vi "FGV_REWORK_destination_selector.vi"(4 "REWORK_commit":refnum<vi>, 6 "REWORK_destination":refnum<vi>, 7 "options":T1, 8 "error_in":errorcluster, 11 "input":variant) -> (0 "error_out":errorcluster, 3 "output":variant)   [LabVIEW 2019]
uses:
  FGV_REWORK_destination_selector.ctl
  _misc/AULocalize/SubVIs/Get Localized Phrase Compact Interface 0D.vi
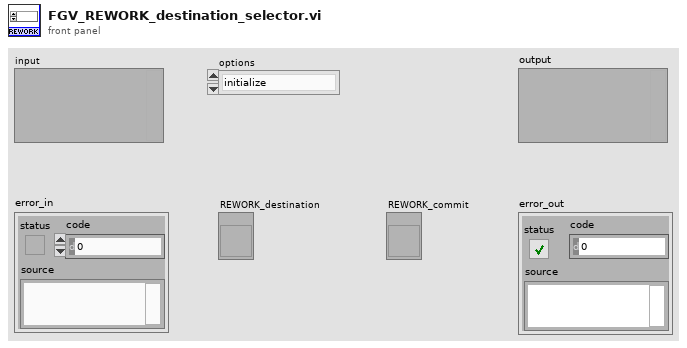
[diagram p1: front panel]
types:
  T1 = typedef "FGV_REWORK_destination_selector.ctl" = enum16{"initialize", "set_values", "display_values", "set_new_login", "enable", "disable", "disable_gray", "get_rework_to", "clear"}
  T2 = enum8{"Enabled", "Disabled", "Disabled and Grayed Out"}
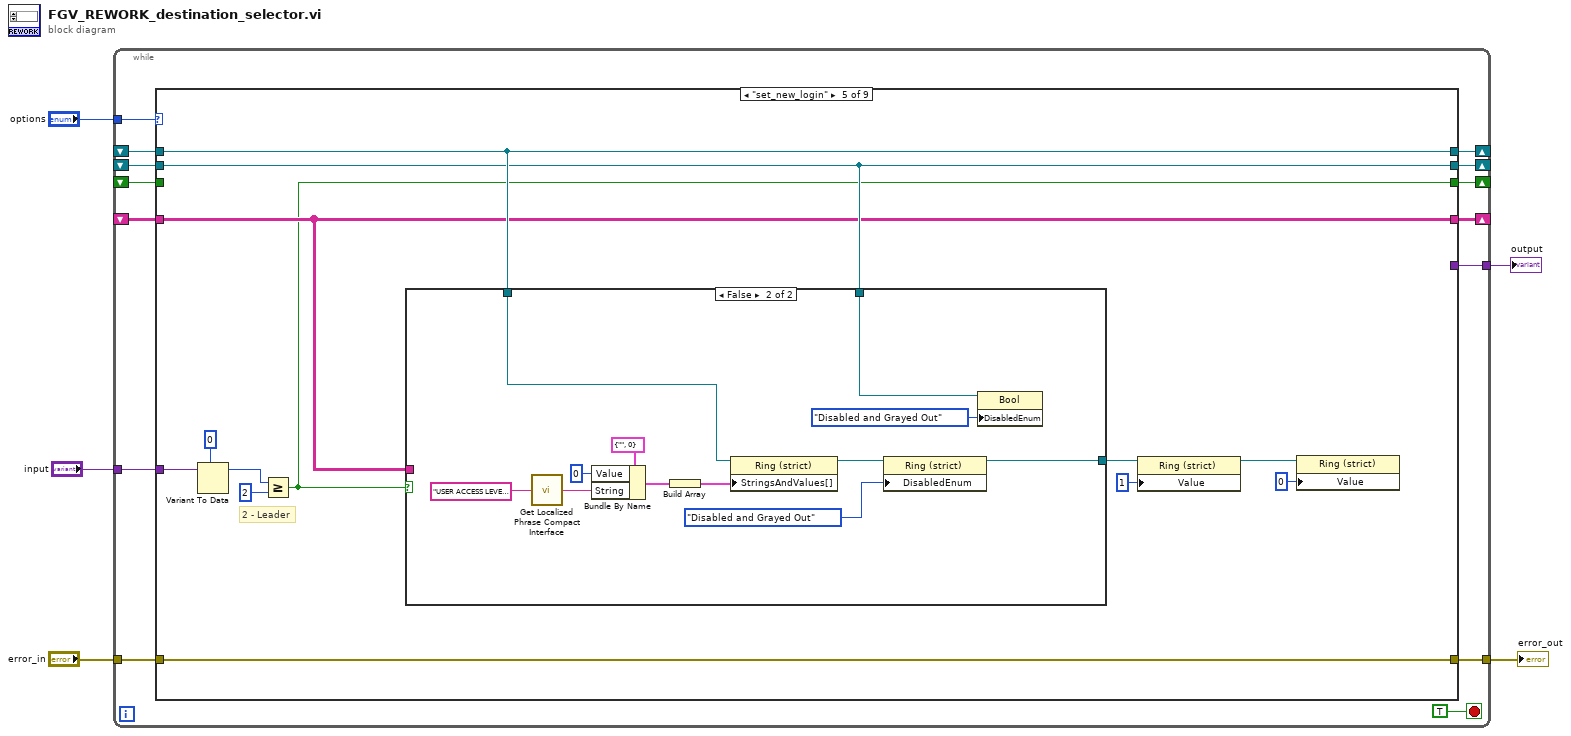
[diagram p0: block diagram]
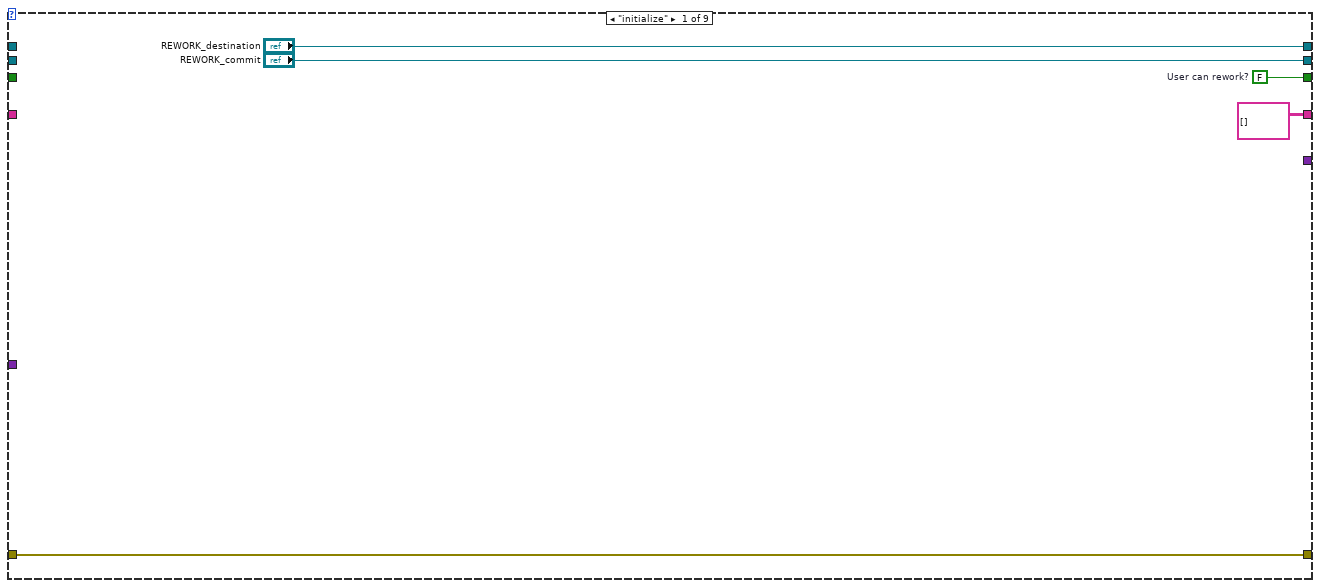
[diagram p2: hidden frame]
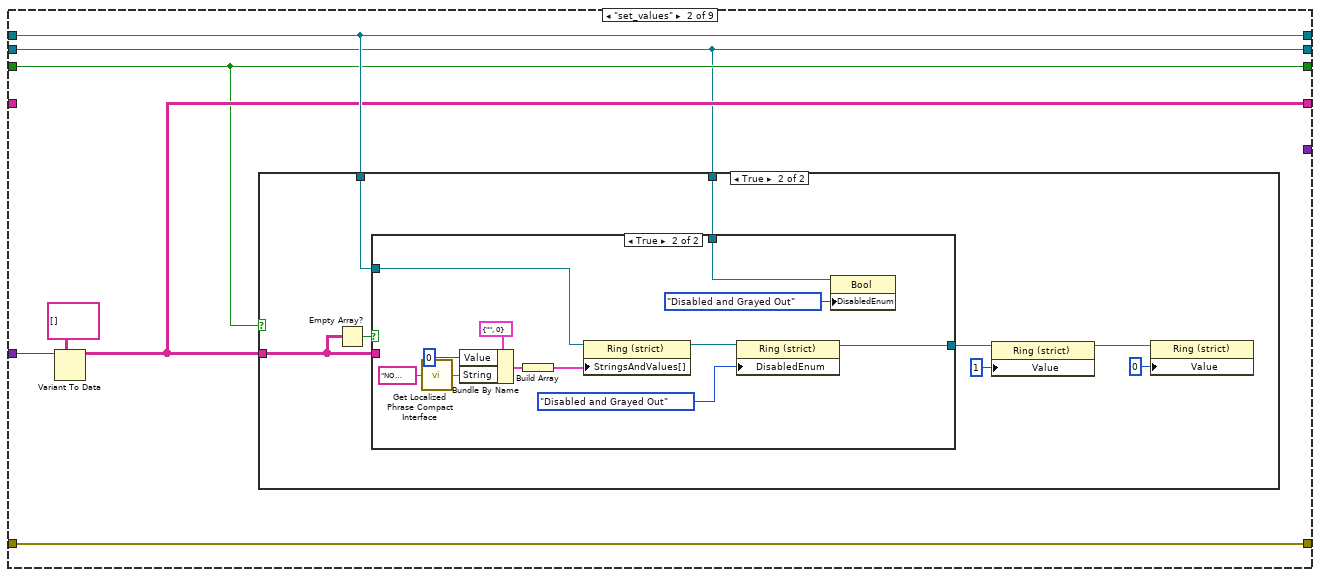
[diagram p3: hidden frame]
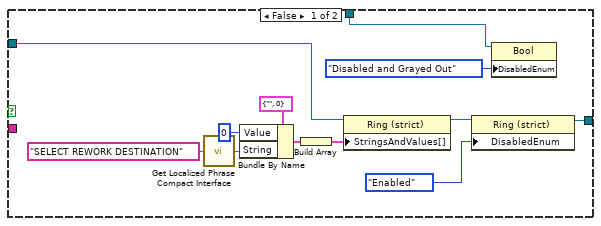
[diagram p5: hidden frame]
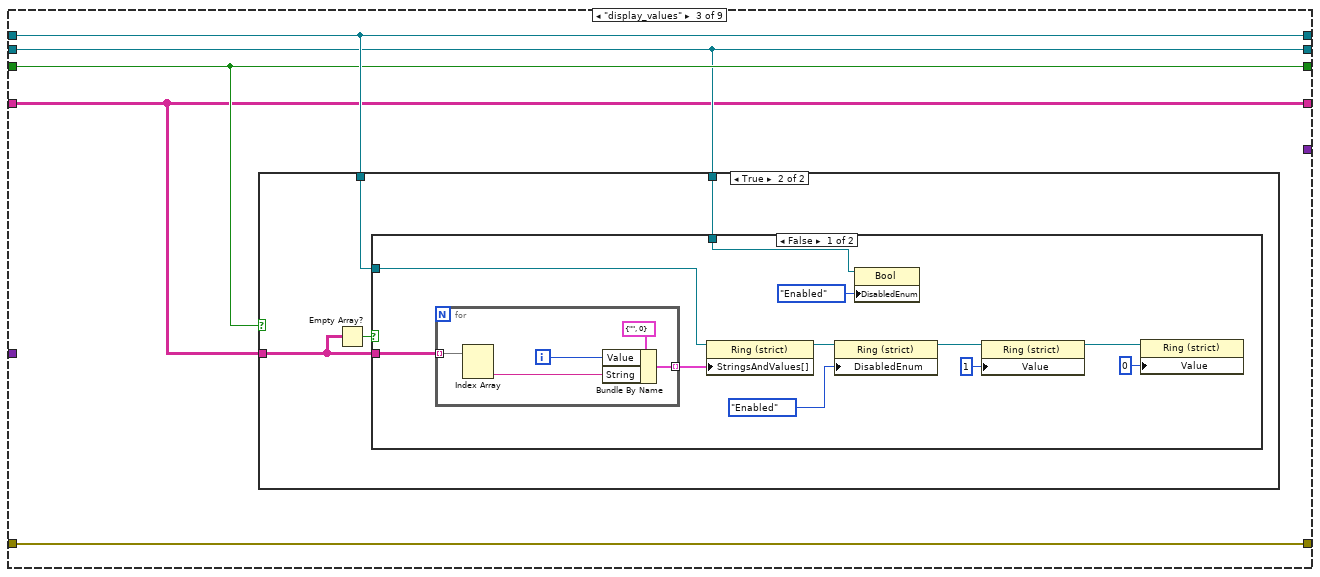
[diagram p6: hidden frame]
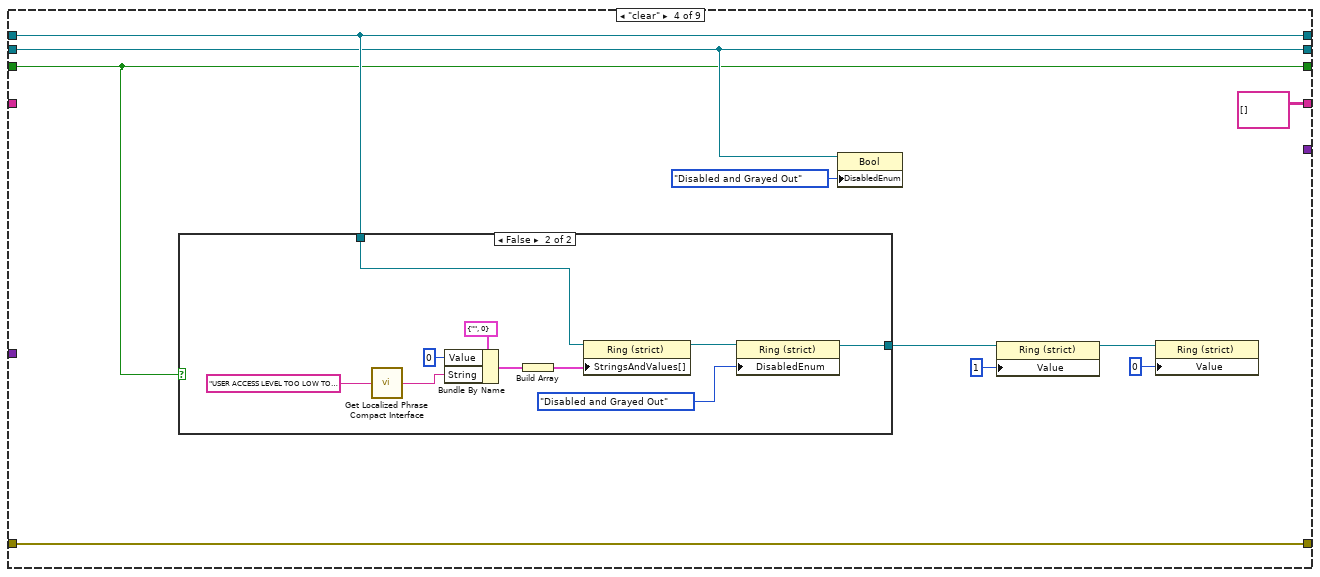
[diagram p9: hidden frame]
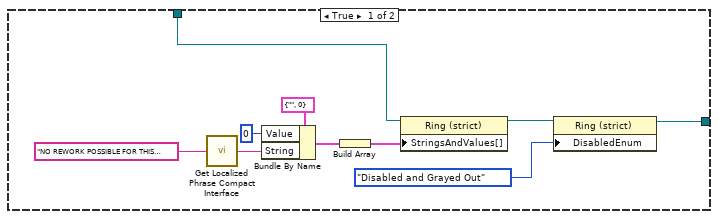
[diagram p10: hidden frame]
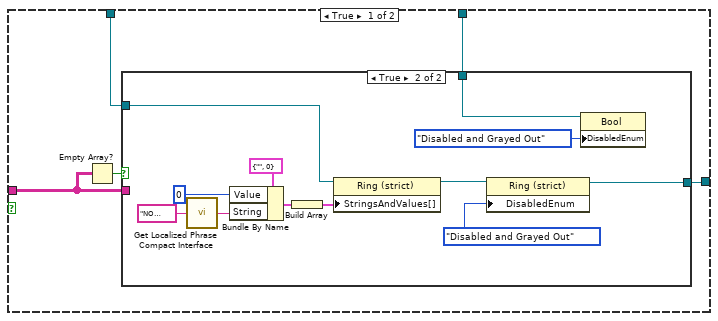
[diagram p11: hidden frame]
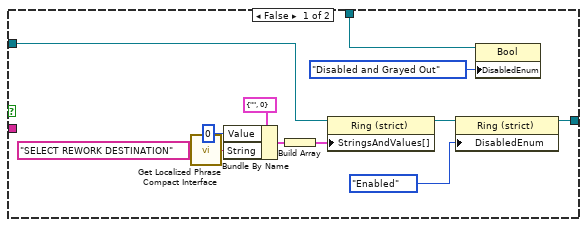
[diagram p12: hidden frame]
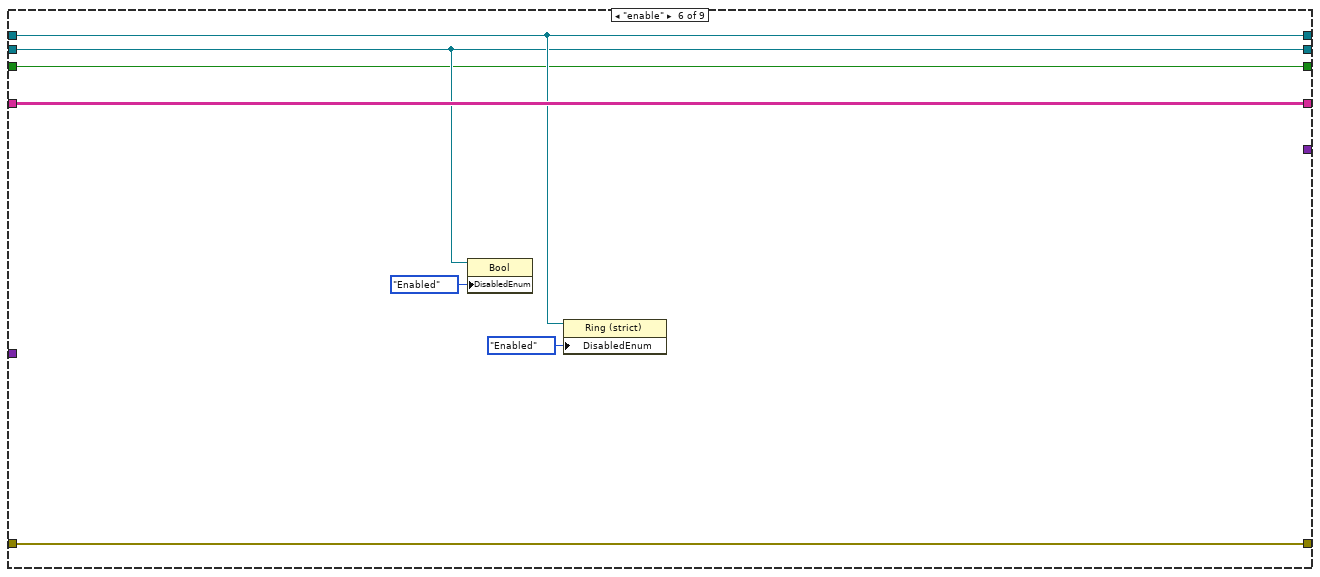
[diagram p13: hidden frame]
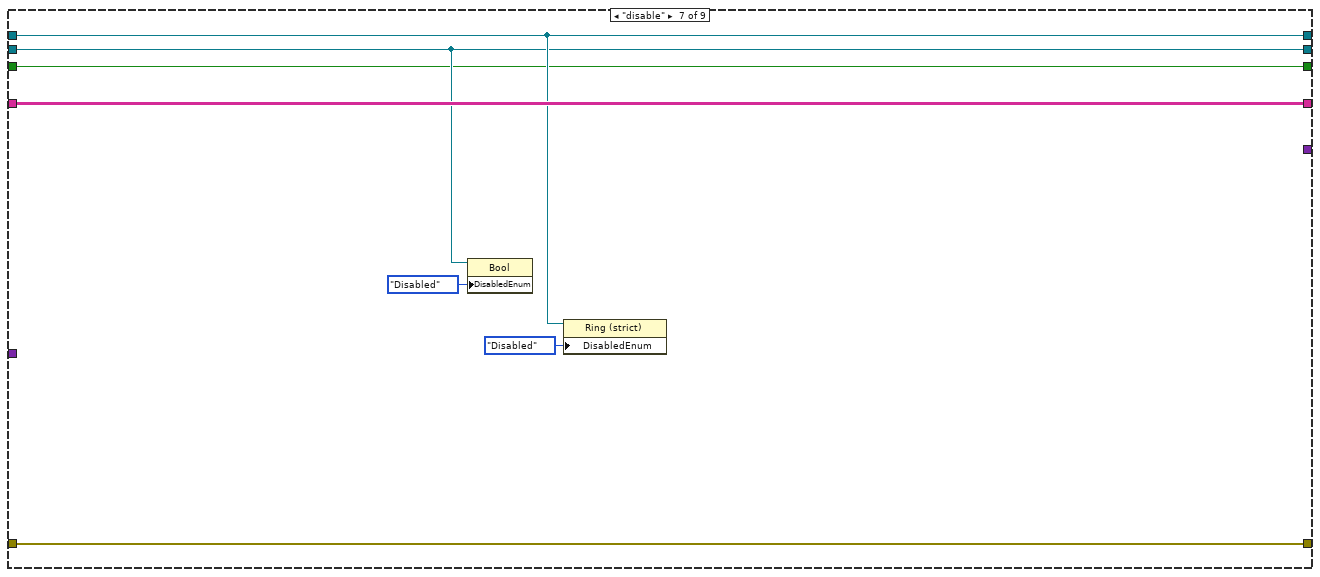
[diagram p14: hidden frame]
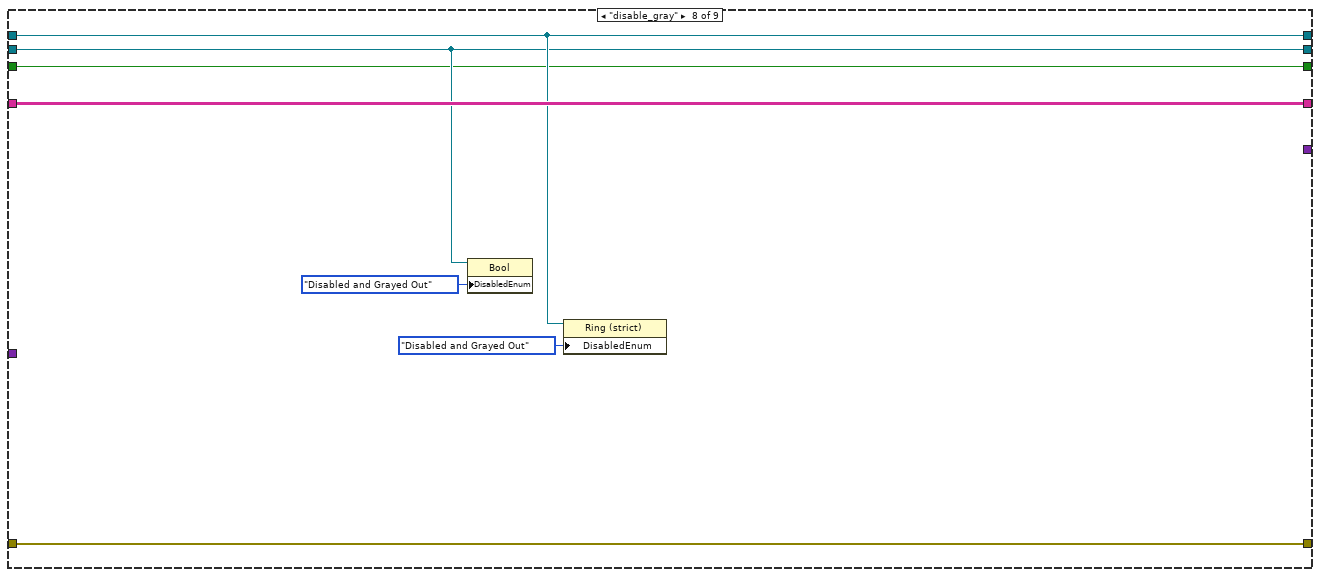
[diagram p15: hidden frame]
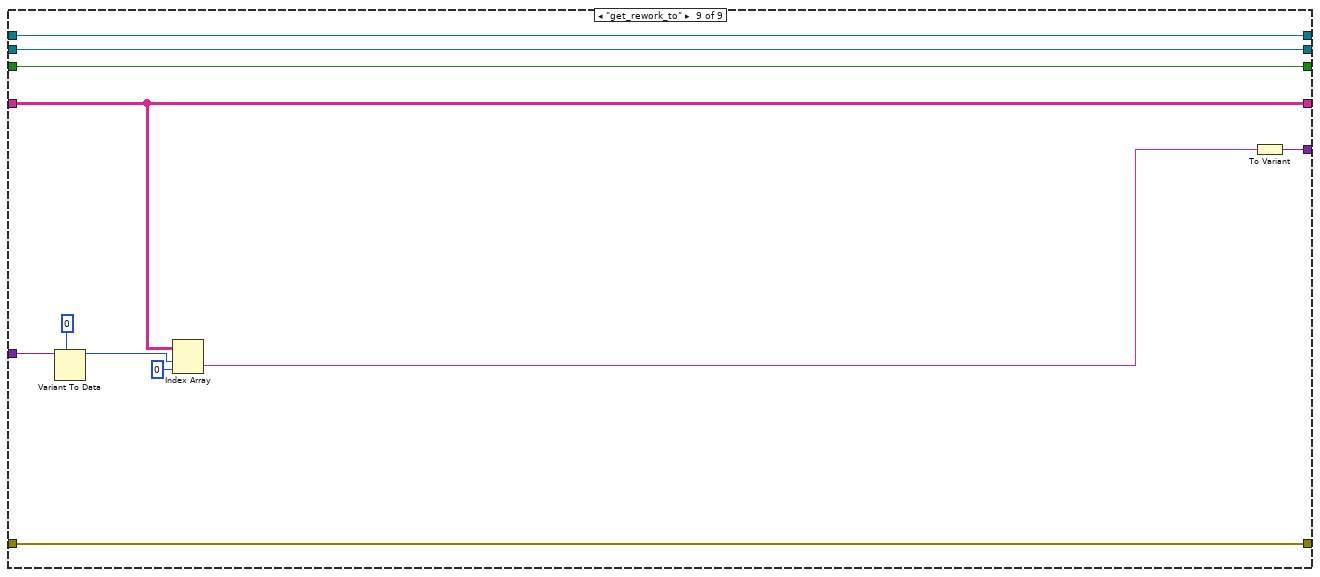
[diagram p16: hidden frame]
diagram:
  n1 = while {
    tunnel: "options" -> [w18]
    tunnel: [w17] -> w5
    tunnel: "error_in" -> [w16]
    shift-right: [w15] -> _
    shift-left: _ -> [w14]
    tunnel: "input" -> [w13]
    shift-right: [w12] -> _
    shift-left: _ -> [w11]
    tunnel: [w10] -> w1
    shift-right: [w9] -> _
    shift-left: _ -> [w8]
    shift-right: [w7] -> _
    shift-left: _ -> [w6]
    stop <- TRUE stop-if-true
    n2 = case shown="\"set_new_login\"" w18 {
      tunnel: [w24 w31 w68 w98 w131 w178 w185 w192 w204] -> w17
      tunnel: w16 -> [w24 w31 w68 w98 w131 w178 w185 w192 w204]
      tunnel: ["REWORK_destination" w30 w67 w97 w130 w175 w182 w189 w203] -> w15
      tunnel: w14 -> [_ w30 w67 w97 w130 w175 w182 w189 w203]
      tunnel: w13 -> [_ w29 _ _ w123 _ _ _ w202]
      tunnel: [string[][] [] ("strings") w27 w64 string[][] [] ("strings") w124 w179 w186 w193 w200] -> w12
      tunnel: w11 -> [_ _ w64 _ w124 w179 w186 w193 w200]
      tunnel: [_ _ _ _ _ _ _ _ w197] -> w10
      tunnel: ["REWORK_commit" w25 w65 w96 w129 w174 w181 w188 w195] -> w9
      tunnel: w8 -> [_ w25 w65 w96 w129 w174 w181 w188 w195]
      tunnel: [w20 w26 w66 w89 w119 w173 w180 w187 w194] -> w7
      tunnel: w6 -> [_ w26 w66 w89 _ w173 w180 w187 w194]
      frame "initialize" {
        w20 = FALSE  # User can rework?
      }
      frame "set_values" {
        n3 = Variant To Data(type=string[][] [] ("strings"), Variant=w29) -> (data=w27:string[][])  [unwired: 1 in, 1 out]
        n4 = case shown="True" w26 {
          tunnel: w30 -> [_ w39]
          tunnel: w27 -> [_ w33]
          tunnel: w25 -> [_ w32]
          frame False {
          }
          frame True {
            n5 = Empty Array?(array=w33) -> (empty?=w34:bool)
            n6 = case shown="True" w34 {
              tunnel: w39 -> [w51 w58]
              tunnel: w33 -> [_ _]
              tunnel: [w47 w55] -> w36
              tunnel: w32 -> [w49 w54]
              frame False {
                n7 = call-poly "Get Localized Phrase Compact Interface.vi"("Key"="SELECT REWORK DESTINATION" ("String")) -> ("Translated Phrase"=w40:string)
                n8 = Bundle By Name(cluster=cluster{"String":string, "Value":u16} {"String"="", "Value"=0}, "Value"=u16 0, "String"=w40) -> (w42:cluster{"String":string, "Value":u16})
                n9 = Build Array(w42) -> (w41:cluster{"String":string, "Value":u16}[])
                n10 = property class="Ring (strict)"(reference=w51, "StringsAndValues[]"=w41) -> (reference out=w48:refnum<vi>)  [unwired: 1 in, 1 out]
                n11 = property class="Ring (strict)"(reference=w48, "DisabledEnum"=T2."Enabled" ("Disabled")) -> (reference out=w47:refnum<vi>)  [unwired: 1 in, 1 out]
                n12 = property class="Bool"(reference=w49, "DisabledEnum"=T2."Disabled and Grayed Out" ("Disabled")) -> ()  [unwired: 1 in, 2 out]
              }
              frame True {
                n13 = call-poly "Get Localized Phrase Compact Interface.vi"("Key"="NO REWORK POSSIBLE FOR THIS GEAR" ("String")) -> ("Translated Phrase"=w52:string)
                n14 = Bundle By Name(cluster=cluster{"String":string, "Value":u16} {"String"="", "Value"=0}, "Value"=u16 0, "String"=w52) -> (w59:cluster{"String":string, "Value":u16})
                n15 = Build Array(w59) -> (w60:cluster{"String":string, "Value":u16}[])
                n16 = property class="Ring (strict)"(reference=w58, "StringsAndValues[]"=w60) -> (reference out=w57:refnum<vi>)  [unwired: 1 in, 1 out]
                n17 = property class="Ring (strict)"(reference=w57, "DisabledEnum"=T2."Disabled and Grayed Out" ("Disabled")) -> (reference out=w55:refnum<vi>)  [unwired: 1 in, 1 out]
                n18 = property class="Bool"(reference=w54, "DisabledEnum"=T2."Disabled and Grayed Out" ("Disabled")) -> ()  [unwired: 1 in, 2 out]
              }
            }
            n19 = property class="Ring (strict)"(reference=w36, "Value"=u16 1) -> (reference out=w35:refnum<vi>)  [unwired: 1 in, 1 out]
            n20 = property class="Ring (strict)"(reference=w35, "Value"=u16 0) -> ()  [unwired: 1 in, 2 out]
          }
        }
      }
      frame "display_values" {
        n21 = case shown="True" w66 {
          tunnel: w67 -> [_ w72]
          tunnel: w64 -> [_ w70]
          tunnel: w65 -> [_ w69]
          frame False {
          }
          frame True {
            n22 = Empty Array?(array=w70) -> (empty?=w71:bool)
            n23 = case shown="False" w71 {
              tunnel: w72 -> [w83 _]
              tunnel: w70 -> [w82 _]
              tunnel: w69 -> [w79 _]
              frame False {
                n24 = for {
                  tunnel: w82 -> [w86] mode=indexing
                  tunnel: [w87] -> w81 mode=indexing
                  i -> [w84]
                  n25 = Index Array(array=w86) -> (element #2=w85:string)  [unwired: 2 in, 1 out]
                  n26 = Bundle By Name(cluster=cluster{"String":string, "Value":u16} {"String"="", "Value"=0}, "Value"=w84, "String"=w85) -> (w87:cluster{"String":string, "Value":u16})
                }
                n27 = property class="Ring (strict)"(reference=w83, "StringsAndValues[]"=w81) -> (reference out=w78:refnum<vi>)  [unwired: 1 in, 1 out]
                n28 = property class="Ring (strict)"(reference=w78, "DisabledEnum"=T2."Enabled" ("Disabled")) -> (reference out=w73:refnum<vi>)  [unwired: 1 in, 1 out]
                n29 = property class="Bool"(reference=w79, "DisabledEnum"=T2."Enabled" ("Disabled")) -> ()  [unwired: 1 in, 2 out]
                n30 = property class="Ring (strict)"(reference=w73, "Value"=u16 1) -> (reference out=w74:refnum<vi>)  [unwired: 1 in, 1 out]
                n31 = property class="Ring (strict)"(reference=w74, "Value"=u16 0) -> ()  [unwired: 1 in, 2 out]
              }
              frame True {
              }
            }
          }
        }
      }
      frame "clear" {
        n32 = case shown="False" w89 {
          tunnel: w97 -> [w108 w118]
          tunnel: [w107 w117] -> w93
          frame True {
            n33 = call-poly "Get Localized Phrase Compact Interface.vi"("Key"="NO REWORK POSSIBLE FOR THIS GEAR" ("String")) -> ("Translated Phrase"=w99:string)
            n34 = Bundle By Name(cluster=cluster{"String":string, "Value":u16} {"String"="", "Value"=0}, "Value"=u16 0, "String"=w99) -> (w102:cluster{"String":string, "Value":u16})
            n35 = Build Array(w102) -> (w103:cluster{"String":string, "Value":u16}[])
            n36 = property class="Ring (strict)"(reference=w108, "StringsAndValues[]"=w103) -> (reference out=w101:refnum<vi>)  [unwired: 1 in, 1 out]
            n37 = property class="Ring (strict)"(reference=w101, "DisabledEnum"=T2."Disabled and Grayed Out" ("Disabled")) -> (reference out=w107:refnum<vi>)  [unwired: 1 in, 1 out]
          }
          frame False {
            n38 = call-poly "Get Localized Phrase Compact Interface.vi"("Key"="USER ACCESS LEVEL TOO LOW TO PERFORM REWORK" ("String")) -> ("Translated Phrase"=w109:string)
            n39 = Bundle By Name(cluster=cluster{"String":string, "Value":u16} {"String"="", "Value"=0}, "Value"=u16 0, "String"=w109) -> (w112:cluster{"String":string, "Value":u16})
            n40 = Build Array(w112) -> (w113:cluster{"String":string, "Value":u16}[])
            n41 = property class="Ring (strict)"(reference=w118, "StringsAndValues[]"=w113) -> (reference out=w111:refnum<vi>)  [unwired: 1 in, 1 out]
            n42 = property class="Ring (strict)"(reference=w111, "DisabledEnum"=T2."Disabled and Grayed Out" ("Disabled")) -> (reference out=w117:refnum<vi>)  [unwired: 1 in, 1 out]
          }
        }
        n43 = property class="Bool"(reference=w96, "DisabledEnum"=T2."Disabled and Grayed Out" ("Disabled")) -> ()  [unwired: 1 in, 2 out]
        n44 = property class="Ring (strict)"(reference=w93, "Value"=u16 1) -> (reference out=w92:refnum<vi>)  [unwired: 1 in, 1 out]
        n45 = property class="Ring (strict)"(reference=w92, "Value"=u16 0) -> ()  [unwired: 1 in, 2 out]
      }
      frame "set_new_login" {
        # "2 - Leader"
        n46 = Variant To Data(type=0 ("y"), Variant=w123) -> (data=w120:i32)  [unwired: 1 in, 1 out]
        n47 = Greater Or Equal?(x=w120, y=2) -> (x >= y?=w119:bool)
        n48 = case shown="False" w119 {
          tunnel: w130 -> [w136 w172]
          tunnel: w124 -> [w134 _]
          tunnel: w129 -> [w133 w171]
          tunnel: [w132 w162] -> w127
          frame True {
            n49 = Empty Array?(array=w134) -> (empty?=w135:bool)
            n50 = case shown="True" w135 {
              tunnel: w136 -> [w138 w155]
              tunnel: w134 -> [_ _]
              tunnel: [w140 w152] -> w132
              tunnel: w133 -> [w139 w151]
              frame False {
                n51 = call-poly "Get Localized Phrase Compact Interface.vi"("Key"="SELECT REWORK DESTINATION" ("String")) -> ("Translated Phrase"=w137:string)
                n52 = Bundle By Name(cluster=cluster{"String":string, "Value":u16} {"String"="", "Value"=0}, "Value"=u16 0, "String"=w137) -> (w147:cluster{"String":string, "Value":u16})
                n53 = Build Array(w147) -> (w148:cluster{"String":string, "Value":u16}[])
                n54 = property class="Ring (strict)"(reference=w138, "StringsAndValues[]"=w148) -> (reference out=w146:refnum<vi>)  [unwired: 1 in, 1 out]
                n55 = property class="Ring (strict)"(reference=w146, "DisabledEnum"=T2."Enabled" ("Disabled")) -> (reference out=w140:refnum<vi>)  [unwired: 1 in, 1 out]
                n56 = property class="Bool"(reference=w139, "DisabledEnum"=T2."Disabled and Grayed Out" ("Disabled")) -> ()  [unwired: 1 in, 2 out]
              }
              frame True {
                n57 = call-poly "Get Localized Phrase Compact Interface.vi"("Key"="NO REWORK POSSIBLE FOR THIS GEAR" ("String")) -> ("Translated Phrase"=w149:string)
                n58 = Bundle By Name(cluster=cluster{"String":string, "Value":u16} {"String"="", "Value"=0}, "Value"=u16 0, "String"=w149) -> (w156:cluster{"String":string, "Value":u16})
                n59 = Build Array(w156) -> (w157:cluster{"String":string, "Value":u16}[])
                n60 = property class="Ring (strict)"(reference=w155, "StringsAndValues[]"=w157) -> (reference out=w154:refnum<vi>)  [unwired: 1 in, 1 out]
                n61 = property class="Ring (strict)"(reference=w154, "DisabledEnum"=T2."Disabled and Grayed Out" ("Disabled")) -> (reference out=w152:refnum<vi>)  [unwired: 1 in, 1 out]
                n62 = property class="Bool"(reference=w151, "DisabledEnum"=T2."Disabled and Grayed Out" ("Disabled")) -> ()  [unwired: 1 in, 2 out]
              }
            }
          }
          frame False {
            n63 = call-poly "Get Localized Phrase Compact Interface.vi"("Key"="USER ACCESS LEVEL TOO LOW TO PERFORM REWORK" ("String")) -> ("Translated Phrase"=w161:string)
            n64 = Bundle By Name(cluster=cluster{"String":string, "Value":u16} {"String"="", "Value"=0}, "Value"=u16 0, "String"=w161) -> (w166:cluster{"String":string, "Value":u16})
            n65 = Build Array(w166) -> (w167:cluster{"String":string, "Value":u16}[])
            n66 = property class="Ring (strict)"(reference=w172, "StringsAndValues[]"=w167) -> (reference out=w165:refnum<vi>)  [unwired: 1 in, 1 out]
            n67 = property class="Ring (strict)"(reference=w165, "DisabledEnum"=T2."Disabled and Grayed Out" ("Disabled")) -> (reference out=w162:refnum<vi>)  [unwired: 1 in, 1 out]
            n68 = property class="Bool"(reference=w171, "DisabledEnum"=T2."Disabled and Grayed Out" ("Disabled")) -> ()  [unwired: 1 in, 2 out]
          }
        }
        n69 = property class="Ring (strict)"(reference=w127, "Value"=u16 1) -> (reference out=w128:refnum<vi>)  [unwired: 1 in, 1 out]
        n70 = property class="Ring (strict)"(reference=w128, "Value"=u16 0) -> ()  [unwired: 1 in, 2 out]
      }
      frame "enable" {
        n71 = property class="Bool"(reference=w174, "DisabledEnum"=T2."Enabled" ("Disabled")) -> ()  [unwired: 1 in, 2 out]
        n72 = property class="Ring (strict)"(reference=w175, "DisabledEnum"=T2."Enabled" ("Disabled")) -> ()  [unwired: 1 in, 2 out]
      }
      frame "disable" {
        n73 = property class="Bool"(reference=w181, "DisabledEnum"=T2."Disabled" ("Disabled")) -> ()  [unwired: 1 in, 2 out]
        n74 = property class="Ring (strict)"(reference=w182, "DisabledEnum"=T2."Disabled" ("Disabled")) -> ()  [unwired: 1 in, 2 out]
      }
      frame "disable_gray" {
        n75 = property class="Bool"(reference=w188, "DisabledEnum"=T2."Disabled and Grayed Out" ("Disabled")) -> ()  [unwired: 1 in, 2 out]
        n76 = property class="Ring (strict)"(reference=w189, "DisabledEnum"=T2."Disabled and Grayed Out" ("Disabled")) -> ()  [unwired: 1 in, 2 out]
      }
      frame "get_rework_to" {
        n77 = Variant To Data(type=u16 0, Variant=w202) -> (data=w198:u16)  [unwired: 1 in, 1 out]
        n78 = Index Array(array=w200, index (row)=w198, index (col)=0 ("disabled index (col)")) -> (element=w196:string)
        n79 = To Variant(anything=w196) -> (Variant=w197:variant)
      }
    }
  }
  "error_out" <- w5
  "output" <- w1
